vi "timer9.vi"(11 "reset":bool) -> (3 "Numeric":dbl=10.671526432037354)   [LabVIEW 2019]
uses:
  Program Files (x86)/National Instruments/LabVIEW 2019/project/EN1Course-master (12)/EN1Course-master/_Subs/SystemLink/SL_Subs/SL_XControl.xctl
  <vilib>/httpClient/POSTBuffer.vi
  Program Files (x86)/National Instruments/LabVIEW 2019/project/EN1Course-master (12)/EN1Course-master/_Subs/SystemLink/SL_Subs/SystemLink_Write_Number.vi
  <vilib>/httpClient/LabVIEWHTTPClient.lvlib
panel:
  in  "timer sec":T1(xcontrol)={"Tag"="Timer", "Type"="U_INT64", "Data"="0"}
  in  "timer min":T1(xcontrol)={"Tag"="Timer1", "Type"="U_INT64", "Data"="0"}
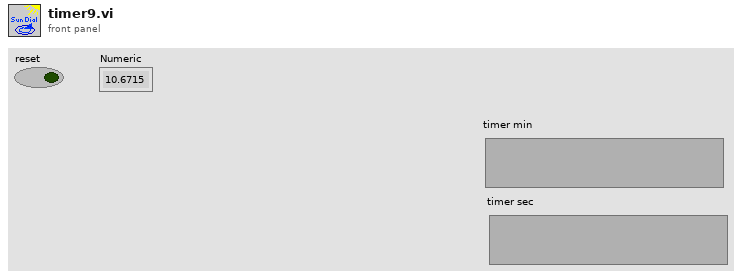
[diagram p1: front panel]
types:
  T1 = cluster{"Tag":string, "Type":string, "Data":string}
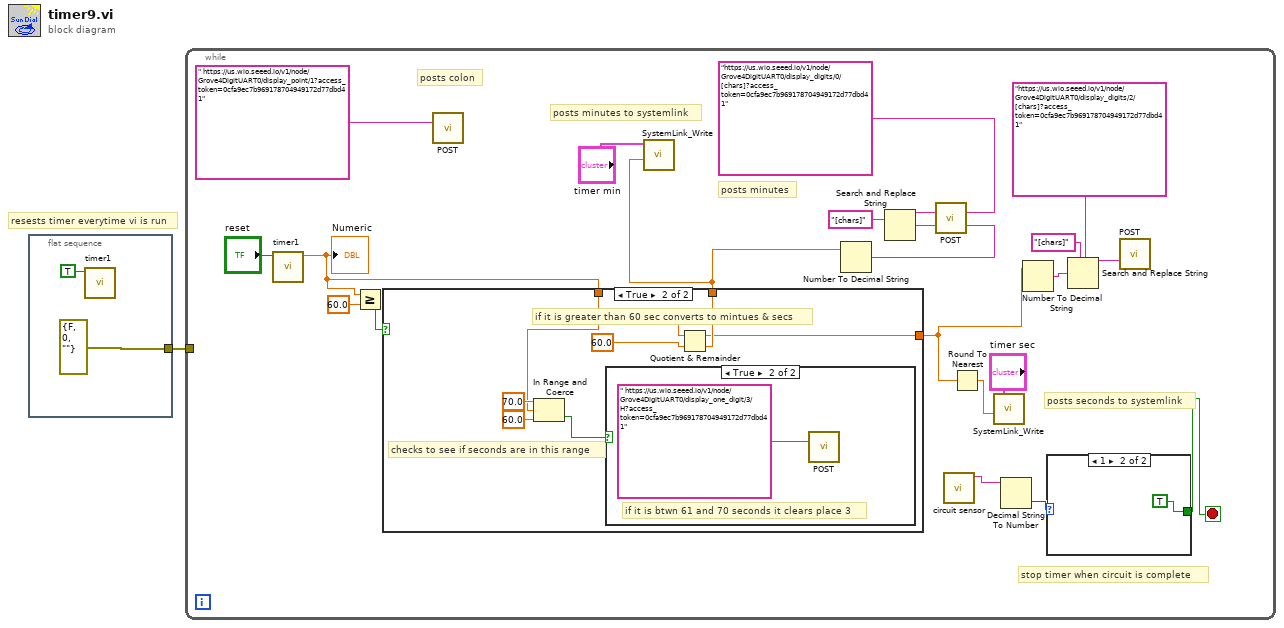
[diagram p0: block diagram]
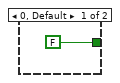
[diagram p2: hidden frame]
diagram:
  # "resests timer everytime vi is run"
  n1 = flat-sequence {
    tunnel: [errorcluster {"status"=FALSE, "code"=0, "source"=""} ("error constant")] -> w1
    frame #0 {
      n2 = call "timer1.vi"("reset"=TRUE ("stop")) -> ()  [unwired: 10 in, 1 out]
    }
  }
  n3 = while {
    tunnel: w1 -> [_]
    stop <- w9 stop-if-true
    # "stop timer when circuit is complete"
    # "posts seconds to systemlink"
    # "posts minutes to systemlink"
    # "posts seconds"
    # "posts minutes"
    # "posts colon"
    n4 = call "timer1.vi"("reset"="reset") -> ("Numeric"=w17:dbl)  [unwired: 10 in]
    "Numeric" <- w17
    n5 = Greater Or Equal?(x=w17, y=60.0) -> (x >= y?=w18:bool)
    n6 = case shown="True" w18 {
      tunnel: w17 -> [w27 w29]
      tunnel: [_ w33] -> w6
      tunnel: [w27 w32] -> w8
      frame False {
        # "if time is under 60 seconds then the format does not change for the timer"
      }
      frame True {
        # "checks to see if seconds are in this range"
        # "if it is greater than 60 sec converts to mintues & secs"
        n7 = In Range and Coerce(upper limit=70.0, x=w29, lower limit=60.0) -> (In Range?=w28:bool)  [unwired: 1 out]
        n8 = case shown="True" w28 {
          frame False {
            # "if it is not between this time the format doesnt change"
          }
          frame True {
            # "if it is btwn 61 and 70 seconds it clears place 3"
            n9 = call-poly <vilib>:"POST.vi"("url"=" https://us.wio.seeed.io/v1/node/Grove4DigitUART0/display_one_digit/3/H?access_token=0cfa9ec7b969178704949172d77dbd41") -> ()  [unwired: 11 in, 4 out]
          }
        }
        n10 = Quotient & Remainder(x=w29, y=60.0) -> (x-y*floor(x/y)=w32:dbl, floor(x/y)=w33:dbl)
      }
    }
    n11 = call-poly <vilib>:"POST.vi"("url"=" https://us.wio.seeed.io/v1/node/Grove4DigitUART0/display_point/1?access_token=0cfa9ec7b969178704949172d77dbd41") -> ()  [unwired: 11 in, 4 out]
    n12 = call-poly "SystemLink_Write.vi"("Numeric"=w6, "SL_XControl"="timer min") -> ()  [unwired: 10 in]
    n13 = Number To Decimal String(number=w6) -> (decimal integer string=w21:string)  [unwired: 1 in]
    n14 = Search and Replace String(input string="https://us.wio.seeed.io/v1/node/Grove4DigitUART0/display_digits/0/[chars]?access_token=0cfa9ec7b969178704949172d77dbd41" ("url"), search string="[chars]", replace string=w21) -> (result string=w24:string)  [unwired: 5 in, 3 out]
    n15 = call-poly <vilib>:"POST.vi"("url"=w24) -> ()  [unwired: 11 in, 4 out]
    n16 = call "circuit sensor.vi"() -> ("Property (str)"=w11:string)  [unwired: 11 in]
    n17 = Round To Nearest(number=w8) -> (nearest integer value=w4:dbl)
    n18 = call-poly "SystemLink_Write.vi"("Numeric"=w4, "SL_XControl"="timer sec") -> ()  [unwired: 10 in]
    n19 = Decimal String To Number(string=w11) -> (number=w10:i32)  [unwired: 2 in, 1 out]
    n20 = Number To Decimal String(number=w8) -> (decimal integer string=w13:string)  [unwired: 1 in]
    n21 = case shown="1" w10 {
      tunnel: [FALSE ("s") TRUE ("s")] -> w9
      frame 0, Default {
      }
      frame 1 {
      }
    }
    n22 = Search and Replace String(input string="https://us.wio.seeed.io/v1/node/Grove4DigitUART0/display_digits/2/[chars]?access_token=0cfa9ec7b969178704949172d77dbd41" ("url"), search string="[chars]", replace string=w13) -> (result string=w16:string)  [unwired: 5 in, 3 out]
    n23 = call-poly <vilib>:"POST.vi"("url"=w16) -> ()  [unwired: 11 in, 4 out]
  }
